vi "PXI Stop AO.vi"   [LabVIEW 2015]
uses:
  PXI Globals.vi
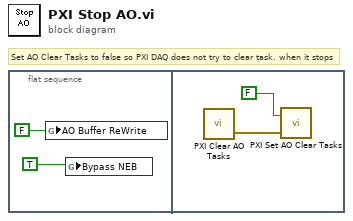
[diagram p0: block diagram]
diagram:
  # "Set AO Clear Tasks to false so PXI DAQ does not try to clear task. when it stops"
  n1 = flat-sequence {
    frame #0 {
      n2 = global write "PXI Globals.vi" "AO Buffer ReWrite"(FALSE) -> ()
      n3 = global write "PXI Globals.vi" "Bypass NEB"(TRUE) -> ()
    }
    frame #1 {
      n4 = call "PXI Clear AO Tasks.vi"() -> ("error out"=w4:errorcluster)  [unwired: 3 in]
      n5 = call "PXI Set AO Clear Tasks.vi"("error in (no error)"=w4, "AO ClearTasks"=FALSE) -> ()  [unwired: 1 in, 1 out]
    }
  }
